vi "Untitled 1.vi"() -> ()   [LabVIEW 2024]
uses:
  <vilib>/picture/picture.llb/imagedata.ctl
panel:
  in  "picture":picture
  out "new picture":picture
  out "image data":T1
  in  "Path":path
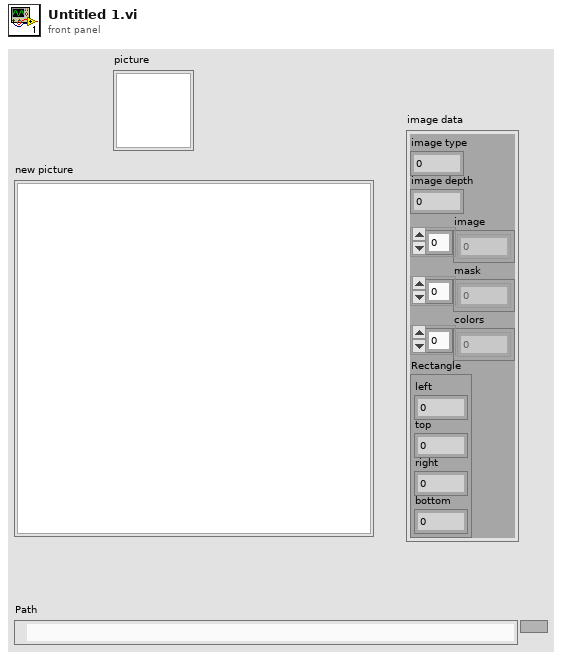
[diagram p1: front panel]
types:
  T1 = typedef "imagedata.ctl" = cluster{"image type":i32, "image depth":i32, "image":u8[], "mask":u8[], "colors":u32[], "Rectangle":cluster{"left":i16, "top":i16, "right":i16, "bottom":i16}}
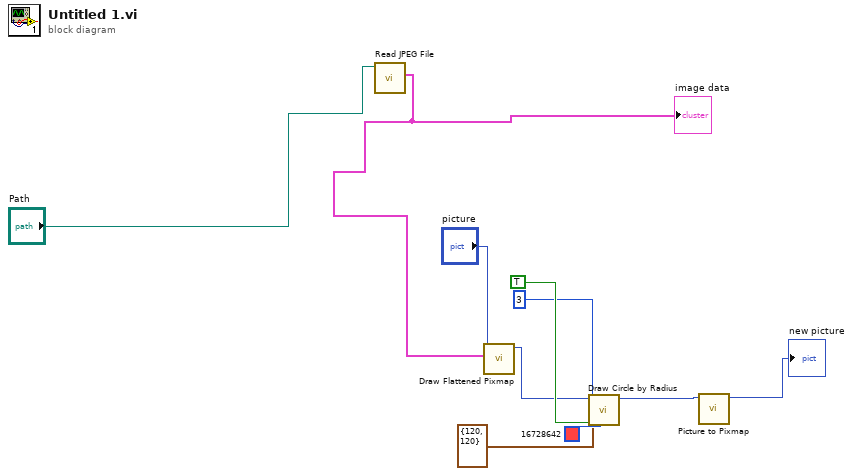
[diagram p0: block diagram]
diagram:
  n1 = call <vilib>:"Read JPEG File.vi"("path to JPEG file"="Path") -> ("image data"=w9:T1)  [unwired: 8 in, 2 out]
  "image data" <- w9
  n2 = call <vilib>:"Draw Flattened Pixmap.vi"("image data"=w9, "picture"="picture") -> ("new picture"=w6:picture)  [unwired: 7 in]
  n3 = call <vilib>:"Draw Circle by Radius.vi"("color(black)"=u32 16728642, "fill?(F)"=TRUE, "pixel center"=cluster{"horizontal":i16, "vertical":i16} {"horizontal"=120, "vertical"=120}, "radius"=i16 3, "picture"=w6) -> ("new picture"=w3:picture)  [unwired: 6 in]
  n4 = call <vilib>:"Picture to Pixmap.vi"("picture"=w3) -> ("new picture"=→"new picture":picture)  [unwired: 9 in, 1 out]
